vi "Ring.vi"() -> ()   [LabVIEW 2019]
panel:
  in  "Rak":u16[][](array[ring])
  in  "s":bool
  out "Ring 2":u16(ring)
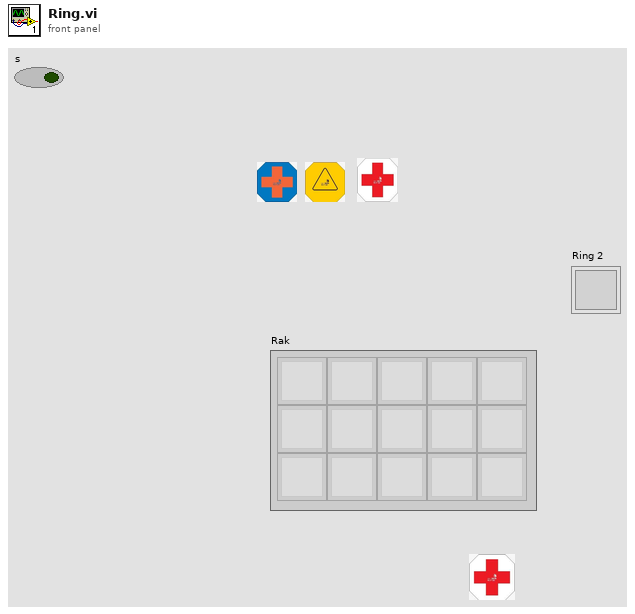
[diagram p1: front panel]
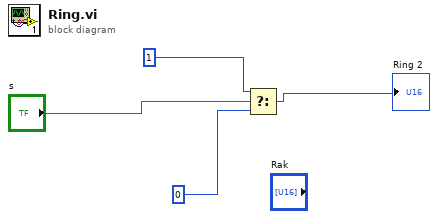
[diagram p0: block diagram]
diagram:
  n1 = Select(t=u16 1 ("Ring"), s="s", f=u16 0) -> (s? t:f=→"Ring 2":u16)
